vi "Self Alias.vi"(11 "TEMPLATE jettl in":refnum<class "TEMPLATE jettl.lvclass">) -> (2 "Self Alias":string)   [LabVIEW 2021, in "_Template.lvlib" / "Templates.lvlib" / "TEMPLATE jettl.lvlib" / "TEMPLATE jettl.lvclass"]
uses:
  TEMPLATE jettl.lvclass
  TEMPLATE jettl.lvclass/TEMPLATE jettl.ctl
  jettl/jettl/jettl/jettl.lvclass
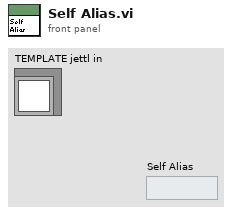
[diagram p1: front panel]
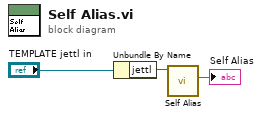
[diagram p0: block diagram]
diagram:
  n1 = Unbundle By Name("TEMPLATE jettl in") -> ("jettl"=w1:refnum<class "jettl.lvclass">)
  n2 = call-dynamic "Self Alias.vi"("jettl in"=w1) -> ("Self Alias"=→"Self Alias":string)  [unwired: 10 in]
